vi "Config Parse Section Helper.vi"(8 "error in":errorcluster, 9 "String In":string) -> (0 "error out":errorcluster, 1 "Key/Value array":cluster{string[], string[]}, 2 "Section Out":string)   [LabVIEW 2017]
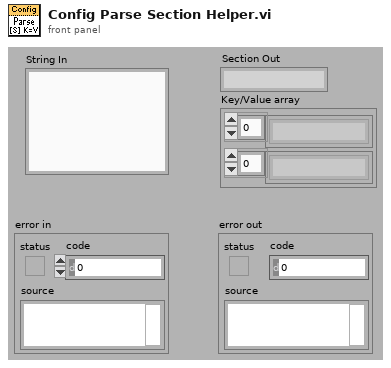
[diagram p1: front panel]
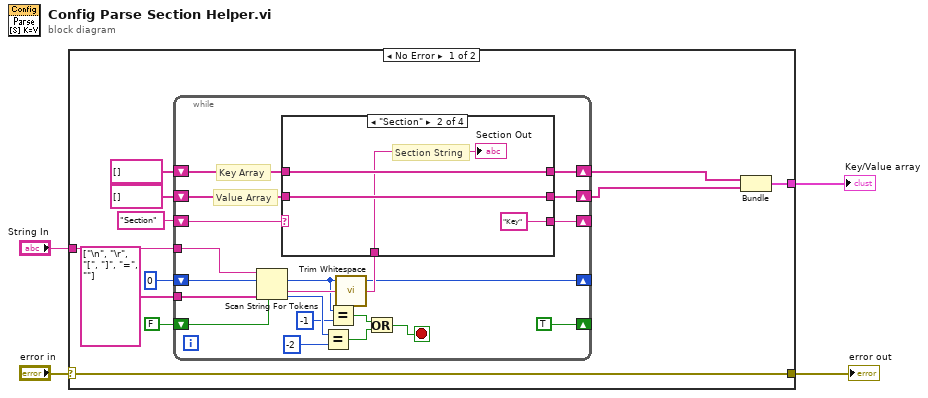
[diagram p0: block diagram]
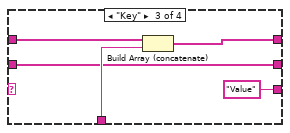
[diagram p3: hidden frame]
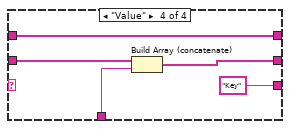
[diagram p4: hidden frame]
diagram:
  n1 = case shown="No Error" "error in" {
    selector: "error in" -> [w8 w52]
    tunnel: [w8 w52] -> w3
    tunnel: "String In" -> [w11 _]
    tunnel: [w6 _] -> w1
    frame No Error {
      n2 = while {
        tunnel: string[] ["\n", "\r", "[", "]", "=", ""] -> [w33]
        shift-right: [TRUE] -> _
        shift-left: FALSE -> [w32]
        shift-right: [w20] -> _
        shift-left: 0 -> [w34]
        shift-right: [w28] -> w5
        shift-left: string[] [] -> [w27]
        shift-right: [w26] -> w7
        shift-left: string[] [] -> [w29]
        shift-right: [w30] -> _
        shift-left: "Section" -> [w31]
        tunnel: w11 -> [w23]
        stop <- w16 stop-if-true
        # "Value Array"
        # "Key Array"
        n3 = Scan String For Tokens(4:w32, 6:w33, 8:w34, 9:w23) -> (0:w24:i32, 1:w21:string, 2:w20:i32)  [unwired: 2 in, 1 out]
        n4 = Equal?(x=w24, y=-2) -> (x = y?=w17:bool)
        n5 = Equal?(x=w20, y=-1) -> (x = y?=w18:bool)
        n6 = call <vilib>:"Trim Whitespace.vi"("string"=w21) -> ("trimmed string"=w22:string)  [unwired: 1 in]
        n7 = case shown="\"Section\"" w31 {
          tunnel: w22 -> [_ w38 w44 w47]
          tunnel: [_ "Key" "Value" "Key"] -> w30
          tunnel: [w37 w40 w45 w50] -> w28
          tunnel: w29 -> [w36 w39 w42 w49]
          tunnel: w27 -> [w37 w40 w43 w50]
          tunnel: [w36 w39 w42 w48] -> w26
          frame Default {
          }
          frame "Section" {
            # "Section String"
            "Section Out" <- w38
          }
          frame "Key" {
            n8 = Build Array (concatenate)(w43, w44) -> (w45:string[])
          }
          frame "Value" {
            n9 = Build Array (concatenate)(w49, w47) -> (w48:string[])
          }
        }
        n10 = Or(x=w18, y=w17) -> (x .or. y?=w16:bool)
      }
      n11 = Bundle(w5, w7) -> (w6:cluster{string[], string[]})  [unwired: 1 in]
    }
    frame Error {
    }
  }
  "error out" <- w3
  "Key/Value array" <- w1
